vi "arrayexp.vi"() -> ()   [LabVIEW 2019]
panel:
  in  "Array 5":bool[](array[boolean])
  out "element 2":dbl
  out "Array 11":dbl[](array[numeric])
  out "Array 10":dbl[](array[numeric])
  out "element":dbl
  out "appended array 3":dbl[](array[numeric])
  out "appended array 2":dbl[][](array[numeric])
  out "appended array":dbl[](array[numeric])
  out "subarray":dbl[](array[numeric])
  out "initialized array 2":dbl[][](array[numeric])
  out "initialized array":dbl[](array[numeric])
  out "size(s) 2":i32[](array[numeric])
  out "size(s)":i32
  in  "1":dbl[][](array[numeric])
  out "2":dbl[][](array[numeric])
  out "Array 9":string[](array[string])
  out "Array 8":bool[](array[boolean])
  out "Array 7":dbl[](array[numeric])
  out "Array 6":string[](array[string])
  out "Array 4":dbl[](array[numeric])
  in  "Array 3":string[](array[string])
  out "Array 2":bool[](array[boolean])
  in  "Array":dbl[](array[numeric])
  out "date/time string":string
  in  "Time Stamp Control":timestamp format="%<%x %.3X>T"
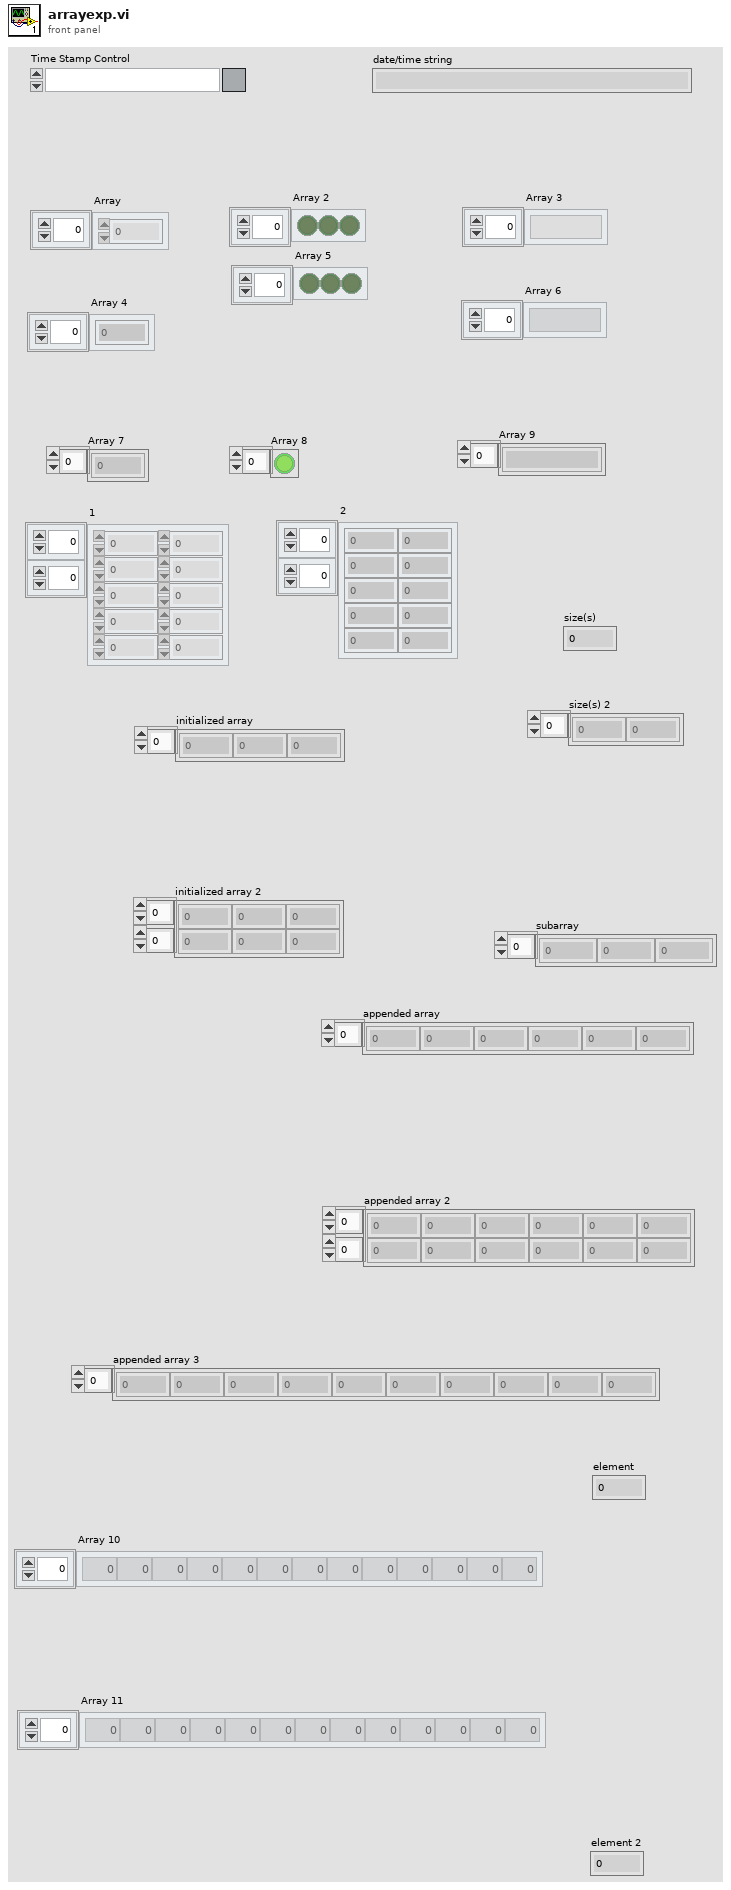
[diagram p1: front panel]
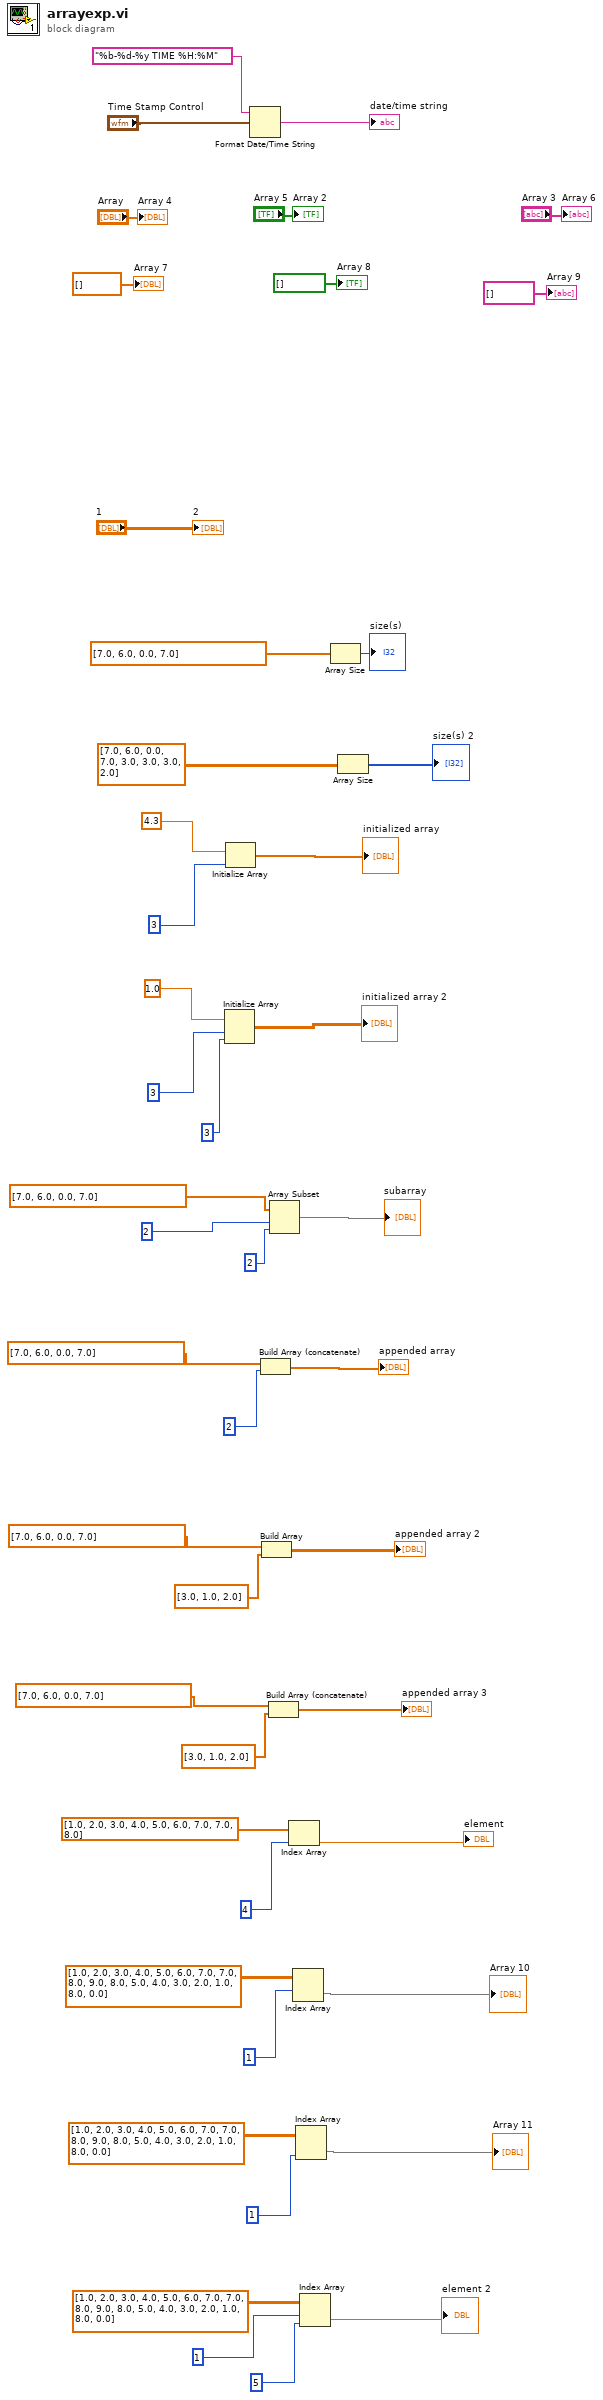
[diagram p0: block diagram]
diagram:
  n1 = Initialize Array(1.0 ("element"), 3 ("dimension size"), 3 ("dimension size")) -> (→"initialized array 2":dbl[][])
  n2 = Initialize Array(4.3 ("element"), 3 ("dimension size")) -> (→"initialized array":dbl[])
  n3 = Format Date/Time String(time format string (%c)="%b-%d-%y TIME %H:%M", seconds (now)="Time Stamp Control") -> (date/time string=→"date/time string":string)  [unwired: 1 in]
  n4 = Build Array (concatenate) "Build Array"(dbl[] [7.0, 6.0, 0.0, 7.0], 2 ("element")) -> (→"appended array":dbl[])
  n5 = Build Array "Build Array"(dbl[] [7.0, 6.0, 0.0, 7.0], dbl[] [3.0, 1.0, 2.0] ("element")) -> (→"appended array 2":dbl[][])
  n6 = Build Array (concatenate) "Build Array"(dbl[] [7.0, 6.0, 0.0, 7.0], dbl[] [3.0, 1.0, 2.0] ("element")) -> (→"appended array 3":dbl[])
  n7 = Array Subset(array=dbl[] [7.0, 6.0, 0.0, 7.0], index=2, length=2) -> (→"subarray":dbl[])
  n8 = Index Array(array=dbl[] [1.0, 2.0, 3.0, 4.0, 5.0, 6.0, 7.0, 7.0, 8.0], index=4) -> (element=→"element":dbl)
  n9 = Index Array(array=dbl[][] [[1.0, 2.0, 3.0, 4.0, 5.0, 6.0, 7.0, 7.0, 8.0], [9.0, 8.0, 5.0, 4.0, 3.0, 2.0, 1.0, 8.0, 0.0]], index (row)=1 ("index")) -> (element=→"Array 10":dbl[])  [unwired: 1 in]
  n10 = Index Array(array=dbl[][] [[1.0, 2.0, 3.0, 4.0, 5.0, 6.0, 7.0, 7.0, 8.0], [9.0, 8.0, 5.0, 4.0, 3.0, 2.0, 1.0, 8.0, 0.0]], index (col)=1 ("index")) -> (element=→"Array 11":dbl[])  [unwired: 1 in]
  n11 = Index Array(array=dbl[][] [[1.0, 2.0, 3.0, 4.0, 5.0, 6.0, 7.0, 7.0, 8.0], [9.0, 8.0, 5.0, 4.0, 3.0, 2.0, 1.0, 8.0, 0.0]], index (row)=1 ("disabled index (row)"), index (col)=5 ("index")) -> (element=→"element 2":dbl)
  n12 = Array Size(array=dbl[] [7.0, 6.0, 0.0, 7.0]) -> (size(s)=→"size(s)":i32)
  n13 = Array Size(array=dbl[][] [[7.0, 6.0, 0.0, 7.0], [3.0, 3.0, 3.0, 2.0]]) -> (size(s)=→"size(s) 2":i32[])
  "Array 2" <- "Array 5"
  "Array 4" <- "Array"
  "Array 6" <- "Array 3"
  "Array 7" <- dbl[] []
  "Array 8" <- bool[] []
  "Array 9" <- string[] []
  "2" <- "1"
